vi "close.vi"(8 "error in (no error)":errorcluster, 11 "NetworkProEM in":refnum<class "Network_ProEm_WinX32.lvclass">) -> (0 "error out":errorcluster)   [LabVIEW 2009, in "Hardware.lvlib" / "HWControllers.lvlib" / "Network_ProEm_WinX32.lvclass"]
uses:
  Network_ProEm_WinX32.lvclass
  NetworkCamera.lvclass
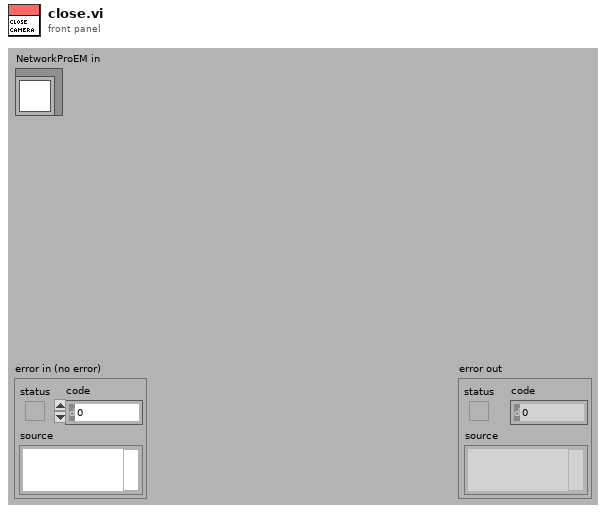
[diagram p1: front panel]
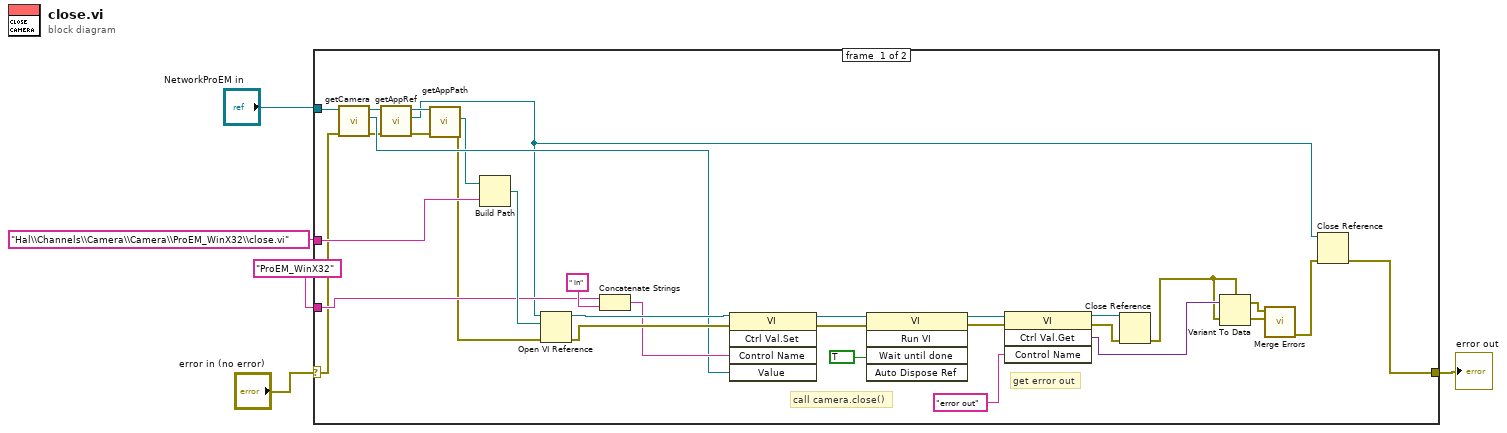
[diagram p0: block diagram]
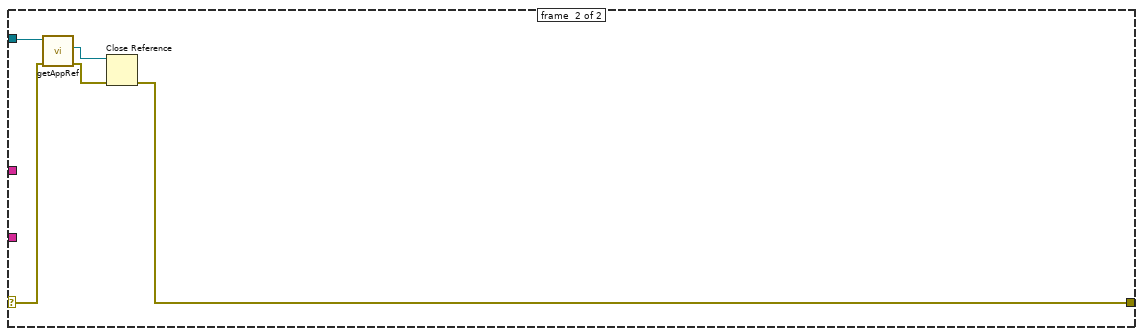
[diagram p2: hidden frame]
diagram:
  n1 = case shown="No Error" "error in (no error)" {
    selector: "error in (no error)" -> [w13 w40]
    tunnel: [w6 w37] -> w1
    tunnel: "NetworkProEM in" -> [w26 w41]
    tunnel: "Hal\\Channels\\Camera\\Camera\\ProEM_WinX32\\close.vi" ("viPath") -> [w30 _]
    tunnel: "ProEM_WinX32" ("Control name") -> [w27 _]
    frame #0 {
      # "get error out"
      # "call camera.close()"
      n2 = call "getCamera.vi"("error in (no error)"=w13, "NetworkCamera in"=w26) -> ("error out"=w15:errorcluster, "Camera"=w23:refnum<class "Camera.lvclass">, "NetworkCamera out"=w25:refnum<class "Network_ProEm_WinX32.lvclass">)  [unwired: 7 in]
      n3 = call "getAppRef.vi"("error in (no error)"=w15, "NetworkCamera in"=w25) -> ("error out"=w14:errorcluster, "appRef"=w7:refnum<vi>, "NetworkCamera out"=w24:refnum<class "Network_ProEm_WinX32.lvclass">)  [unwired: 7 in]
      n4 = call "getAppPath.vi"("error in (no error)"=w14, "NetworkCamera in"=w24) -> ("error out"=w12:errorcluster, "appPath"=w22:path)  [unwired: 7 in, 1 out]
      n5 = Build Path(base path=w22, name or relative path=w30) -> (appended path=w36:path)
      n6 = Open VI Reference(application reference (local)=w7, vi path=w36, error in (no error)=w12) -> (vi reference=w32:refnum<vi>, error out=w31:errorcluster)  [unwired: 3 in]
      n7 = Concatenate Strings(w27, " in") -> (w28:string)
      n8 = invoke class="VI" method="Ctrl Val.Set"(reference=w32, error in=w31, "Control Name"=w28, "Value"=w23) -> (reference out=w35:refnum<vi>, error out=w34:errorcluster)  [unwired: 1 in, 3 out]
      n9 = invoke class="VI" method="Run VI"(reference=w35, error in=w34, "Wait until done"=TRUE) -> (reference out=w10:refnum<vi>, error out=w9:errorcluster)  [unwired: 2 in, 3 out]
      n10 = invoke class="VI" method="Ctrl Val.Get"(reference=w10, error in=w9, "Control Name"="error out") -> (reference out=w21:refnum<vi>, error out=w20:errorcluster, "Get Control Value Variant"=w19:variant)  [unwired: 1 in, 1 out]
      n11 = Close Reference(reference=w21, error in (no error)=w20) -> (error out=w11:errorcluster)
      n12 = Variant To Data(error in=w11, Variant=w19, type=w11) -> (error out=w18:errorcluster, data=w17:errorcluster)
      n13 = call <vilib>:"Merge Errors.vi"("error in 2 (no error)"=w18, "error in 1 (no error)"=w17) -> ("error out"=w8:errorcluster)  [unwired: 5 in]
      n14 = Close Reference(reference=w7, error in (no error)=w8) -> (error out=w6:errorcluster)
    }
    frame #1 {
      n15 = call "getAppRef.vi"("error in (no error)"=w40, "NetworkCamera in"=w41) -> ("error out"=w38:errorcluster, "appRef"=w39:refnum<vi>)  [unwired: 7 in, 1 out]
      n16 = Close Reference(reference=w39, error in (no error)=w38) -> (error out=w37:errorcluster)
    }
  }
  "error out" <- w1
